vi "Read Control Parameters.vi"(8 "error in (no error)":errorcluster, 11 "Lakeshore 336 in":refnum<class "Lakeshore 336.lvclass">) -> (0 "error out":errorcluster, 2 "Control Parameters":cluster{"P":dbl, "I":dbl, "D":u16}[](array[cluster]), 3 "Lakeshore 336 out":refnum<class "Lakeshore 336.lvclass">)   [LabVIEW 2022 SP3, in "Lakeshore 336.lvclass"]
uses:
  Lakeshore 336.lvclass
  Lakeshore 336.lvclass/Lakeshore 336.ctl
  Temp Control.lvclass
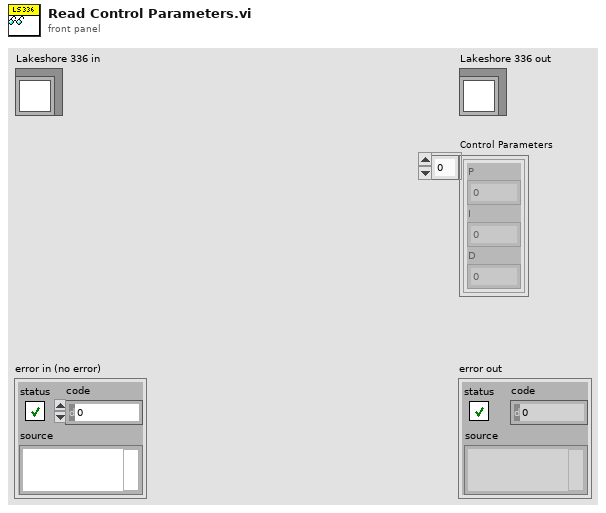
[diagram p1: front panel]
types:
  T1 = typedef "Lakeshore 336.lvclass/Lakeshore 336 Channel Settings cluster.ctl" = cluster{"Input (0:None)":u16, "Power Up Enable (F: Off)":bool, "Mode (0:Off)":u16, "Max Current (0:User Specified)":u16, "Heater Out Display (1:Current)":u16, "Max User Current (2.000)":dbl, "Heater Resistance (1:25 Ohms)":u16, "PID":T2, "Name":string}
  T2 = typedef "Lakeshore 336.lvclass/Lakeshore 336 PID cluster.ctl" = cluster{"P":dbl, "I":dbl, "D":dbl}
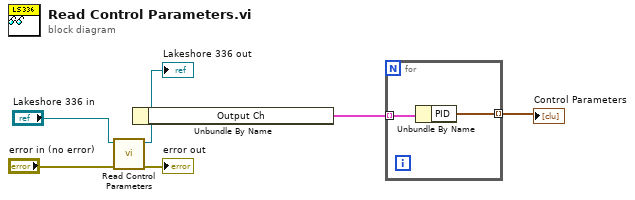
[diagram p0: block diagram]
diagram:
  n1 = call-parent "Read Control Parameters.vi"("error in (no error)"="error in (no error)", "Temp Control in"="Lakeshore 336 in") -> ("error out"=→"error out":errorcluster, "Temp Control out"=w3:refnum<class "Lakeshore 336.lvclass">)  [unwired: 7 in, 1 out]
  "Lakeshore 336 out" <- w3
  n2 = Unbundle By Name(w3) -> ("Output Ch"=w2:T1[])
  n3 = for {
    tunnel: w2 -> [w8] mode=indexing
    tunnel: [w7] -> w1 mode=indexing
    n4 = Unbundle By Name(w8) -> ("PID"=w7:T2)
  }
  "Control Parameters" <- w1
